vi "Init Events.vi"(8 "error in (no error)":errorcluster, 11 "SB App in":refnum<class "SB App.lvclass">) -> (0 "error out":errorcluster, 3 "SB App out":refnum<class "SB App.lvclass">)   [LabVIEW 2020, in "SB App.lvlib" / "SB App.lvclass"]
uses:
  SB App.lvclass
  Board Size Update.ctl
  Game Start Data.ctl
  Start Position Data.ctl
  SquareBattle/Team ID.ctl
  SquareBattle/Position.ctl
  SB App.lvclass/SB App.ctl
  SB App.lvlib
  SquareBattle/SquareBattle.lvlib
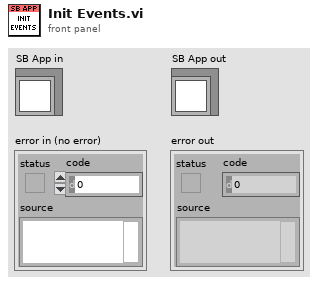
[diagram p1: front panel]
types:
  T1 = typedef "SquareBattle.lvlib/Team ID.ctl" = u32
  T2 = typedef "SB App.lvlib/Start Position Data.ctl" = cluster{"Team ID":T1, "Position":T3}
  T3 = typedef "SquareBattle.lvlib/Position.ctl" = cluster{"Row":i32, "Col":i32}
  T4 = typedef "SB App.lvlib/Game Start Data.ctl" = cluster{"NA":bool}
  T5 = typedef "SB App.lvlib/Board Size Update.ctl" = cluster{"Board Size":i32}
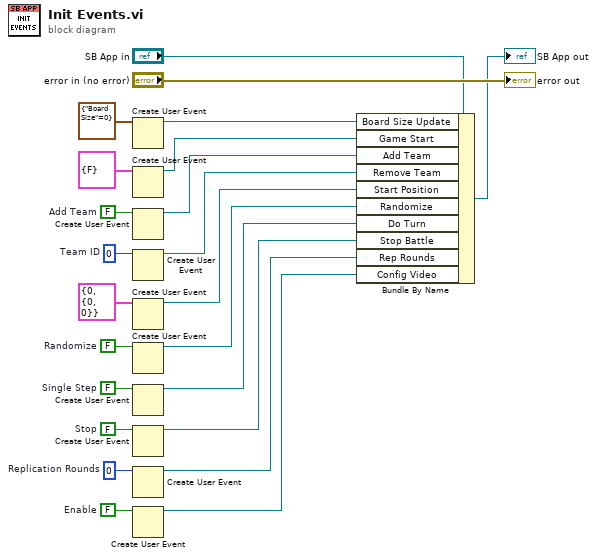
[diagram p0: block diagram]
diagram:
  w2 = FALSE  # Enable
  w4 = u32 0  # Replication Rounds
  w6 = T1 0  # Team ID
  w8 = FALSE  # Stop
  w10 = FALSE  # Single Step
  w12 = FALSE  # Randomize
  w16 = FALSE  # Add Team
  n1 = Create User Event(user event datatype=T5 {"Board Size"=0} ("Board Size Update")) -> (user event=w19:refnum<user-event>)  [unwired: 1 in, 1 out]
  n2 = Create User Event(user event datatype=T4 {"NA"=FALSE} ("Game Start Data")) -> (user event=w17:refnum<user-event>)  [unwired: 1 in, 1 out]
  n3 = Create User Event(user event datatype=w16) -> (user event=w15:refnum<user-event>)  [unwired: 1 in, 1 out]
  n4 = Create User Event(user event datatype=w6) -> (user event=w5:refnum<user-event>)  [unwired: 1 in, 1 out]
  n5 = Create User Event(user event datatype=T2 {"Team ID"=0, "Position"={"Row"=0, "Col"=0}} ("Start Position Data")) -> (user event=w13:refnum<user-event>)  [unwired: 1 in, 1 out]
  n6 = Create User Event(user event datatype=w12) -> (user event=w11:refnum<user-event>)  [unwired: 1 in, 1 out]
  n7 = Create User Event(user event datatype=w10) -> (user event=w9:refnum<user-event>)  [unwired: 1 in, 1 out]
  n8 = Create User Event(user event datatype=w8) -> (user event=w7:refnum<user-event>)  [unwired: 1 in, 1 out]
  n9 = Create User Event(user event datatype=w4) -> (user event=w3:refnum<user-event>)  [unwired: 1 in, 1 out]
  n10 = Create User Event(user event datatype=w2) -> (user event=w1:refnum<user-event>)  [unwired: 1 in, 1 out]
  n11 = Bundle By Name(cluster="SB App in", "Board Size Update"=w19, "Game Start"=w17, "Add Team"=w15, "Remove Team"=w5, "Start Position"=w13, "Randomize"=w11, "Do Turn"=w9, "Stop Battle"=w7, "Rep Rounds"=w3, "Config Video"=w1) -> (→"SB App out":refnum<class "SB App.lvclass">)
  "error out" <- "error in (no error)"
